vi "MU Write Params.vi"(8 "error in (no error)":errorcluster, 10 "verify":bool, 11 "handle":u64) -> (0 "error out (no error)":errorcluster, 2 "valid":bool[](array[boolean]), 3 "function return":u32)   [LabVIEW 2017, in "MU_3SL_interface.lvlib"]
uses:
  MU_3SL_interface.lvlib
  lib/MU_3SL_interface.dll
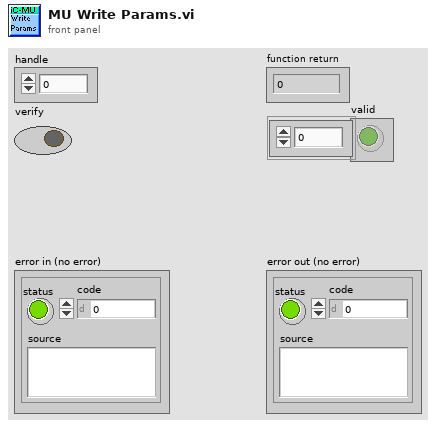
[diagram p1: front panel]
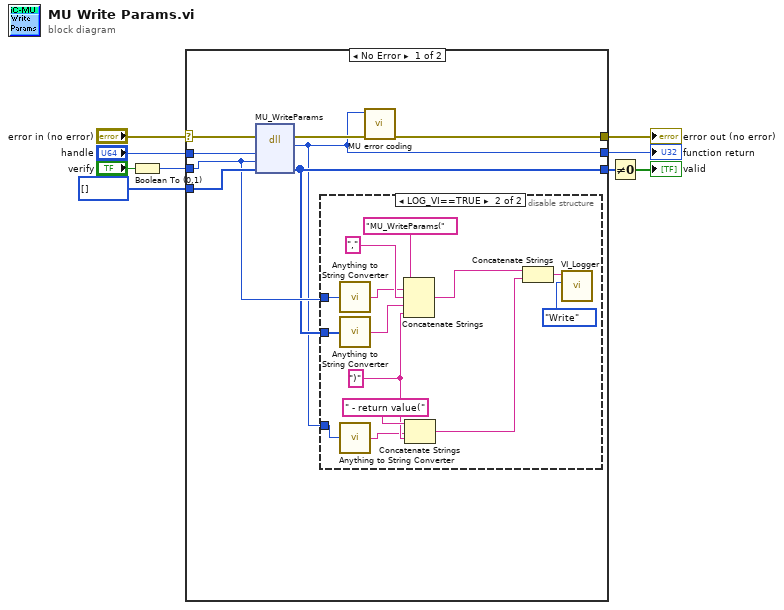
[diagram p0: block diagram]
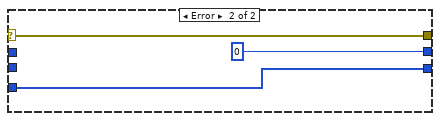
[diagram p3: hidden frame]
diagram:
  n1 = Boolean To (0,1)(Boolean="verify") -> (0, 1=w4:i16)
  n2 = case shown="No Error" "error in (no error)" {
    selector: "error in (no error)" -> [w14 w34]
    tunnel: [w10 u32 0 ("return type")] -> w9
    tunnel: "handle" -> [w17 _]
    tunnel: [w15 w34] -> w7
    tunnel: w4 -> [w12 _]
    tunnel: u8[] [] ("valid") -> [w13 w32]
    tunnel: [w11 w32] -> w2
    frame No Error {
      n3 = dll-call lib="C:/Users/bes/AppData/Roaming/work/mu_9so/icsubmodules/soft_mu_3sl_master/lv_interface/lib/MU_3SL_interface**.*" fn="MU_WriteParams"(error in=w14, "handle"=w17, "verify"=w12, "valid"=w13) -> (error out=w16:errorcluster, "return type"=w10:u32, "valid"=w11:u8[])  [unwired: 4 in, 1 out]
      n4 = disable-structure shown="LOG_VI==TRUE" {
        disable-tunnel: w10 -> [_ w24]
        disable-tunnel: w12 -> [_ w20]
        disable-tunnel: w11 -> [_ w19]
        frame condition #0 {
        }
        frame condition #1 (active) {
          w25 = ")" ("string")
          n5 = call "Anything to String Converter.vi"("anything"=w20) -> ("String"=w21:string)
          n6 = call "Anything to String Converter.vi"("anything"=w19) -> ("String"=w22:string)
          n7 = call "Anything to String Converter.vi"("anything"=w24) -> ("String"=w23:string)
          n8 = Concatenate Strings("MU_WriteParams(" ("Info in"), w21, "," ("string"), w22, w25) -> (w18:string)
          n9 = Concatenate Strings(" - return value(" ("string"), w23, w25) -> (w29:string)
          n10 = Concatenate Strings(w18, w29) -> (w28:string)
          n11 = call "VI_Logger.vi"("Action (Read)"=enum16{"Write", "Read"}."Write", "Info in"=w28) -> ()  [unwired: 8 in, 2 out]
        }
      }
      n12 = call "MU error coding.vi"("error in (no error)"=w16, "function return in"=w10) -> ("error out"=w15:errorcluster)  [unwired: 9 in]
    }
    frame Error {
    }
  }
  "function return" <- w9
  "error out (no error)" <- w7
  n13 = Not Equal To 0?(x=w2) -> (x != 0?=→"valid":bool[])
